vi "Create Get Destroy.vi"(8 "error In":errorcluster, 11 "State (Get)":T1=enum."Get") -> (0 "Error Out":errorcluster, 3 "Ref":refnum<user-event>)   [LabVIEW 2018, in "GUI.lvclass"]
uses:
  GUI.lvclass
  User Event State.ctl
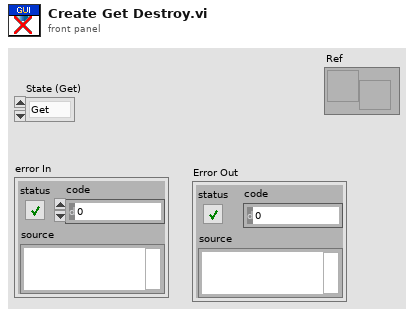
[diagram p1: front panel]
types:
  T1 = typedef "GUI.lvclass/User Event State.ctl" = enum16{"Create", "Get", "Destroy"}
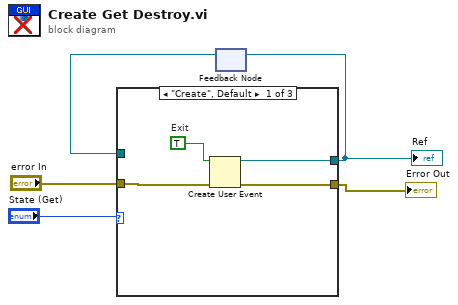
[diagram p0: block diagram]
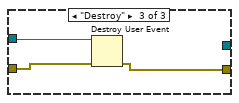
[diagram p3: hidden frame]
diagram:
  n1 = feedback #1() -> (w3:refnum<user-event>)  [unwired: 1 in]
  n2 = case shown="\"Create\", Default" "State (Get)" {
    tunnel: "error In" -> [w9 w10 w14]
    tunnel: [w8 w11 _] -> w2
    tunnel: w3 -> [_ w11 w13]
    tunnel: [w7 w10 w12] -> w1
    frame "Create", Default {
      w6 = TRUE  # Exit
      n3 = Create User Event(user event datatype=w6, error in=w9) -> (user event=w8:refnum<user-event>, error out=w7:errorcluster)
    }
    frame "Get" {
    }
    frame "Destroy" {
      n4 = Destroy User Event(user event=w13, error in=w14) -> (error out=w12:errorcluster)
    }
  }
  "Error Out" <- w1
  "Ref" <- w2
  n5 = feedback-in #1(w2) -> ()
